vi "Initialize Shared Variables.vi"(8 "error in (no error)":errorcluster, 9 "Access":T2={"Read Access"=enum."None", "Write Access"=enum."Allowed"}, 10 "Channel Type Array":T3[](array[typedef]), 11 "Shared Variable Array":string[](array[string])) -> (0 "error out":errorcluster, 3 "Shared Variable Cluster":T1)   [LabVIEW 2012, in "Shared Variable Custom Device.lvlib"]
uses:
  Shared Variable Custom Device.lvlib
  <vilib>/Utility/VariantDataType/Type.ctl
  Shared Variable Cluster.ctl
  <vilib>/Utility/VariantDataType/VariantType.lvlib
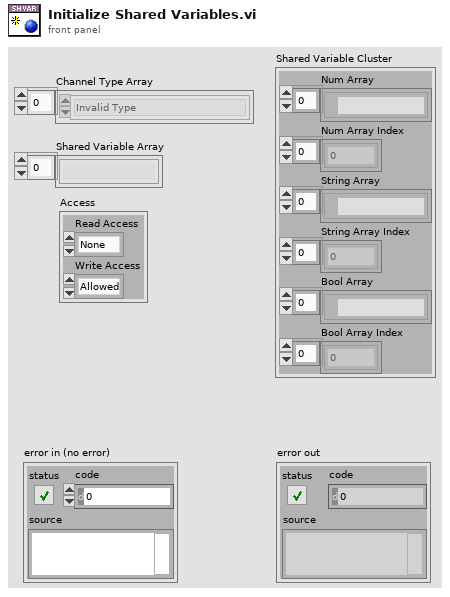
[diagram p1: front panel]
types:
  T1 = typedef "Shared Variable Custom Device.lvlib/Shared Variable Cluster.ctl" = cluster{"Num Array":refnum<k21>[], "Num Array Index":i32[], "String Array":refnum<k21>[], "String Array Index":i32[], "Bool Array":refnum<k21>[], "Bool Array Index":i32[]}
  T2 = cluster{"Read Access":enum8{"Allowed", "Required", "None"}, "Write Access":enum8{"Allowed", "Required", "None"}}
  T3 = typedef "VariantType.lvlib/Type.ctl" = enum8{"Invalid Type", "Void", "I8", "I16", "I32", "I64", "U8", "U16", "U32", "U64", "Single Float", "Double Float", "Extended Float", "Single Complex", "Double Complex", "Extended Complex", "Enum U8", "Enum U16", "Enum U32", "Enum U64", "Single Float With Unit", "Double Float With Unit", "Extended Float With Unit", "Single Complex with Unit", "Double Complex with Unit", "Extended Complex with Unit", "Boolean", "String", "Path", "Picture", "Tag", "Array", "Cluster", "Variant", "LV Variant", "Waveform", "Timestamp", "Digital Waveform", "Digital Data", "ExpressData", "Refnum", "External Data", "VI", "Poly VI", "LabVIEW Class Instance", "Fixed Point"}
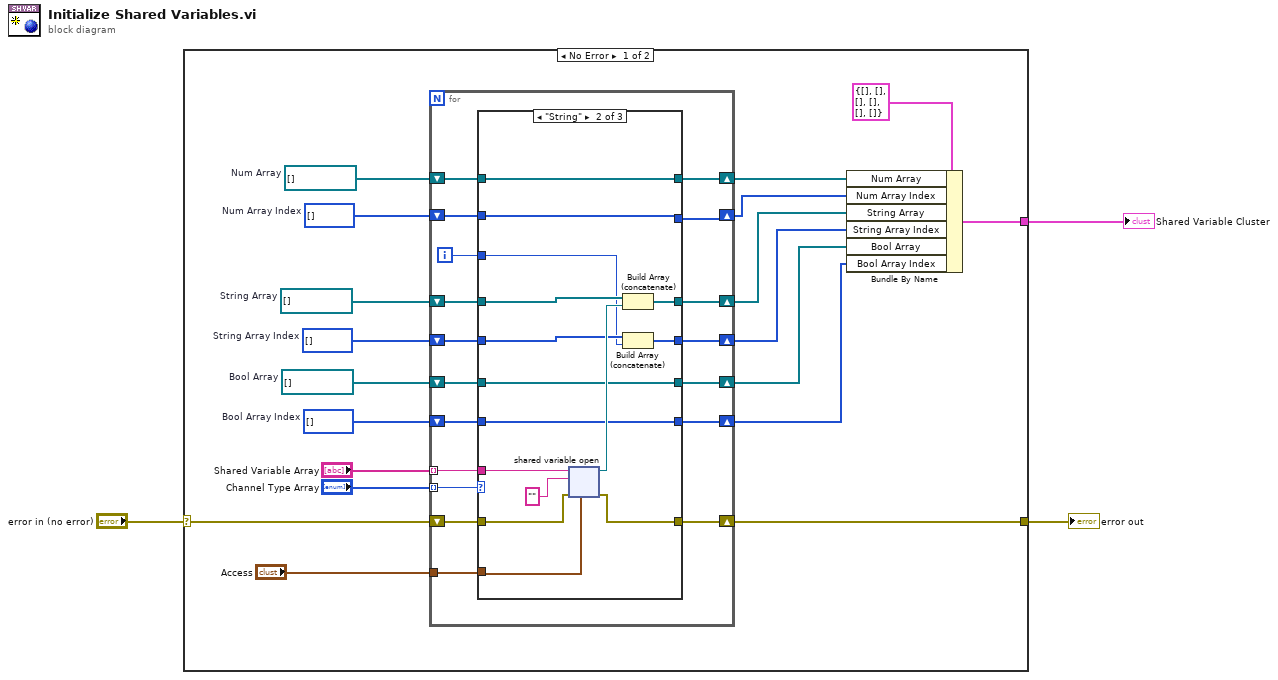
[diagram p0: block diagram]
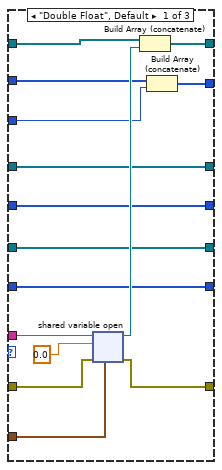
[diagram p2: hidden frame]
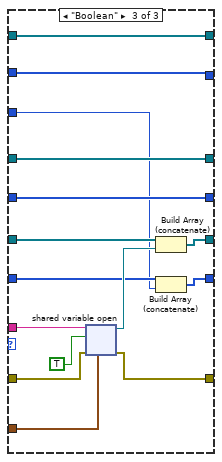
[diagram p3: hidden frame]
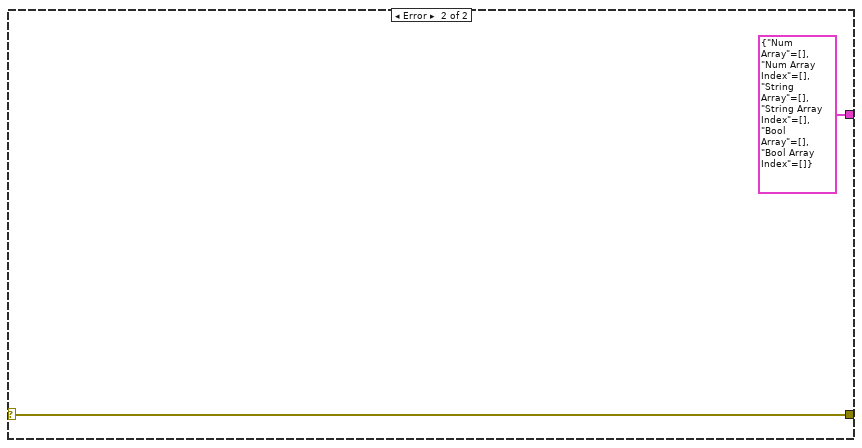
[diagram p4: hidden frame]
diagram:
  n1 = case shown="No Error" "error in (no error)" {
    selector: "error in (no error)" -> [w5 w87]
    tunnel: [w6 T1 {"Num Array"=[], "Num Array Index"=[], "String Array"=[], "String Array Index"=[], "Bool Array"=[], "Bool Array Index"=[]}] -> w3
    tunnel: [w4 w87] -> w1
    frame No Error {
      w14 = i32[] []  # Bool Array Index
      w15 = refnum<k21>[] []  # Bool Array
      w16 = i32[] []  # String Array Index
      w17 = refnum<k21>[] []  # String Array
      w18 = i32[] []  # Num Array Index
      w22 = refnum<k21>[] []  # Num Array
      n2 = for {
        tunnel: "Shared Variable Array" -> [w39] mode=indexing
        tunnel: "Channel Type Array" -> [w40] mode=indexing
        tunnel: "Access" -> [w38]
        shift-right: [w36] -> w13
        shift-left: w22 -> [w37]
        shift-right: [w33] -> w11
        shift-left: w18 -> [w35]
        shift-right: [w31] -> w10
        shift-left: w17 -> [w32]
        shift-right: [w29] -> w9
        shift-left: w16 -> [w30]
        shift-right: [w27] -> w8
        shift-left: w15 -> [w28]
        shift-right: [w25] -> w7
        shift-left: w14 -> [w26]
        shift-right: [w23] -> w4
        shift-left: w5 -> [w24]
        i -> [w34]
        n3 = case shown="\"String\"" w40 {
          tunnel: w39 -> [w55 w68 w81]
          tunnel: w38 -> [w53 w66 w79]
          tunnel: w37 -> [w52 w70 w85]
          tunnel: [w50 w70 w85] -> w36
          tunnel: w35 -> [w49 w69 w84]
          tunnel: w34 -> [w48 w61 w74]
          tunnel: [w47 w69 w84] -> w33
          tunnel: w32 -> [w46 w65 w83]
          tunnel: [w46 w64 w83] -> w31
          tunnel: w30 -> [w45 w62 w82]
          tunnel: [w45 w60 w82] -> w29
          tunnel: w28 -> [w44 w59 w78]
          tunnel: [w44 w59 w76] -> w27
          tunnel: w26 -> [w43 w58 w75]
          tunnel: [w43 w58 w73] -> w25
          tunnel: w24 -> [w42 w57 w72]
          tunnel: [w41 w56 w71] -> w23
          frame "Double Float", Default {
            n4 = shared-variable-open(w55, w42, 0.0, w53) -> (w51:refnum<k21>, w41:errorcluster)
            n5 = Build Array (concatenate)(w52, w51) -> (w50:refnum<k21>[])
            n6 = Build Array (concatenate)(w49, w48) -> (w47:i32[])
          }
          frame "String" {
            n7 = shared-variable-open(w68, w57, "" ("String"), w66) -> (w63:refnum<k21>, w56:errorcluster)
            n8 = Build Array (concatenate)(w65, w63) -> (w64:refnum<k21>[])
            n9 = Build Array (concatenate)(w62, w61) -> (w60:i32[])
          }
          frame "Boolean" {
            n10 = shared-variable-open(w81, w72, TRUE, w79) -> (w77:refnum<k21>, w71:errorcluster)
            n11 = Build Array (concatenate)(w78, w77) -> (w76:refnum<k21>[])
            n12 = Build Array (concatenate)(w75, w74) -> (w73:i32[])
          }
        }
      }
      n13 = Bundle By Name(cluster=T1 {"Num Array"=[], "Num Array Index"=[], "String Array"=[], "String Array Index"=[], "Bool Array"=[], "Bool Array Index"=[]}, "Num Array"=w13, "Num Array Index"=w11, "String Array"=w10, "String Array Index"=w9, "Bool Array"=w8, "Bool Array Index"=w7) -> (w6:T1)
    }
    frame Error {
    }
  }
  "Shared Variable Cluster" <- w3
  "error out" <- w1
